vi "Write plugin VI Refs.vi"(8 "error in (no error)":errorcluster, 10 "plugin VI Refs":refnum<vi>[](array[refnum])=[refnum], 11 "subpanel (abstract) in":refnum<class "subpanel (abstract).lvclass">) -> (0 "error out":errorcluster, 3 "subpanel (abstract) out":refnum<class "subpanel (abstract).lvclass">)   [LabVIEW 2023, in "GUI.lvlib" / "subpanel (abstract).lvclass"]
uses:
  subpanel (abstract).lvclass
  subpanel (abstract).lvclass/subpanel (abstract).ctl
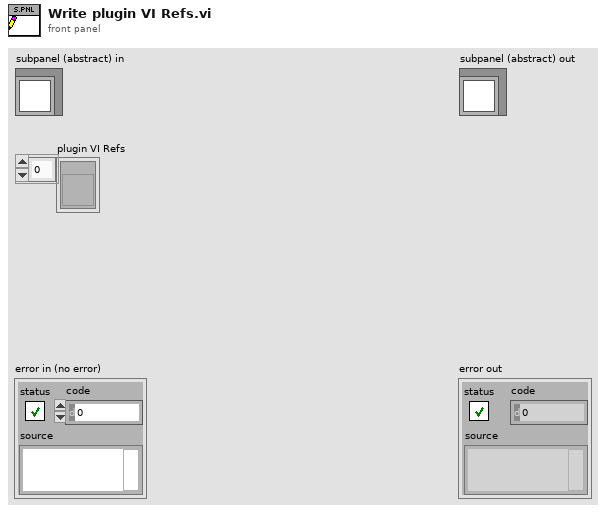
[diagram p1: front panel]
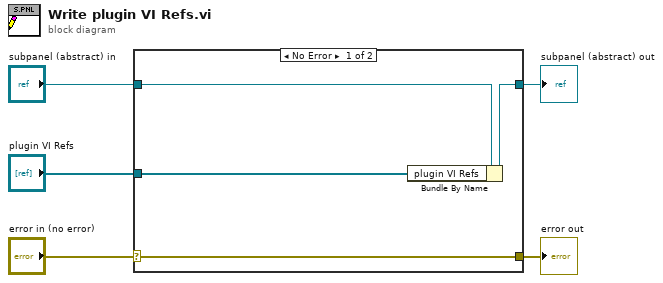
[diagram p0: block diagram]
diagram:
  n1 = case shown="No Error" "error in (no error)" {
    selector: "error in (no error)" -> [w9 w10]
    tunnel: [w9 w10] -> w4
    tunnel: [w7 w11] -> w2
    tunnel: "subpanel (abstract) in" -> [w8 w11]
    tunnel: "plugin VI Refs" -> [w6 _]
    frame No Error {
      n2 = Bundle By Name(cluster=w8, "plugin VI Refs"=w6) -> (w7:refnum<class "subpanel (abstract).lvclass">)
    }
    frame Error {
    }
  }
  "error out" <- w4
  "subpanel (abstract) out" <- w2
